vi "Agilent Fetch.vi"() -> ()   [LabVIEW 2009]
panel:
  out "error out":errorcluster
  in  "VISA resource name":refnum<visa-resource-name>
  out "Output Data":string[](array[string])
  in  "Numbers Only (T:On)":bool=TRUE
  out "Output Data (Numbers Only)":dbl[](array[numeric]) format="%.2e"
  out "Error Message":string
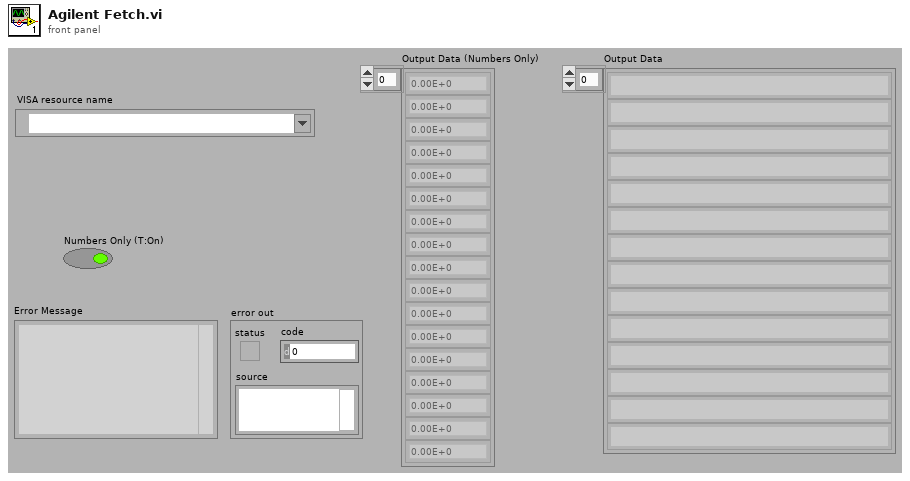
[diagram p1: front panel]
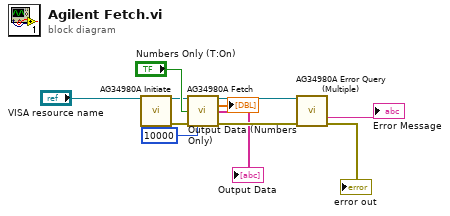
[diagram p0: block diagram]
diagram:
  n1 = call "AG34980A Initiate.vi"("VISA resource name"="VISA resource name") -> ("VISA resource name out"=w7:refnum<visa-resource-name>, "error out"=w5:errorcluster)  [unwired: 13 in]
  n2 = call "AG34980A Fetch.vi"("VISA resource name"=w7, "Numbers Only (T:On)"="Numbers Only (T:On)", "error in (no error)"=w5, "Byte Count (1024 bytes)"=10000) -> ("VISA resource name out"=w8:refnum<visa-resource-name>, "Output Data (Numbers Only)"=→"Output Data (Numbers Only)":dbl[], "Output Data"=→"Output Data":string[], "error out"=w6:errorcluster)  [unwired: 7 in, 1 out]
  n3 = call "AG34980A Error Query (Multiple).vi"("VISA resource name"=w8, "error in (no error)"=w6) -> ("Error Message"=→"Error Message":string, "error out"=→"error out":errorcluster)  [unwired: 10 in, 2 out]
